vi "DAQ.Get Number of Channels from Channel String.vi"(3 "Channels String":string="PXI1Slot2/ai1:3") -> (1 "# channels":i32)   [LabVIEW 2019, in "Instrument.Lockin.lvlib" / "Instrument.DAQ.lvclass"]
uses:
  Instrument.DAQ.lvclass
panel:
  out "names out":string[](array[string])
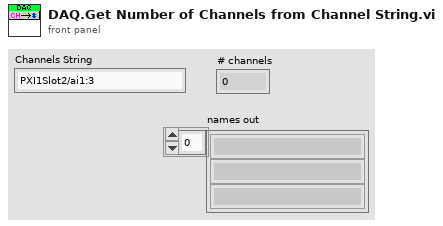
[diagram p1: front panel]
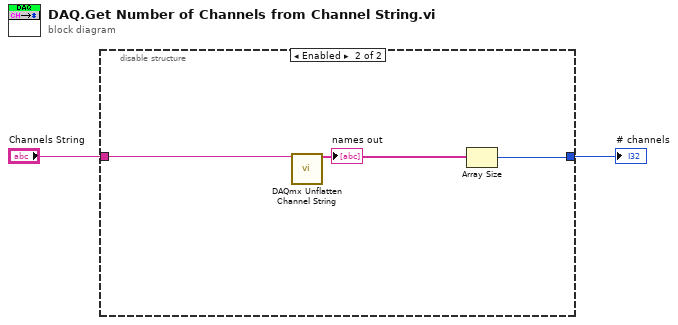
[diagram p0: block diagram]
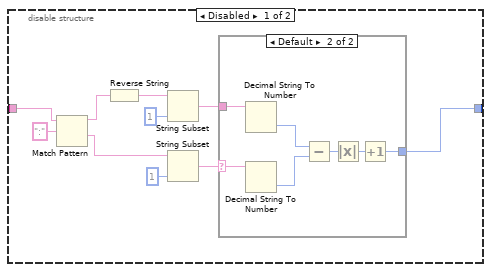
[diagram p2: hidden frame]
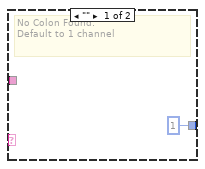
[diagram p3: hidden frame]
diagram:
  n1 = disable-structure shown="Enabled" {
    disable-tunnel: [w5 w21] -> w2
    disable-tunnel: "Channels String" -> [w3 w23]
    frame Disabled {
      n2 = Match Pattern(string=w3, regular expression=":") -> (before substring=w7:string, after substring=w8:string)  [unwired: 1 in, 2 out]
      n3 = Reverse String(1:w7) -> (0:w6:string)
      n4 = String Subset(string=w6, length (rest)=1 ("length (rest)")) -> (substring=w9:string)  [unwired: 1 in]
      n5 = String Subset(string=w8, length (rest)=1 ("length (rest)")) -> (substring=w4:string)  [unwired: 1 in]
      n6 = case shown="Default" w4 {
        selector: w4 -> [_ w17]
        tunnel: w9 -> [_ w20]
        tunnel: [1 w18] -> w5
        frame "" {
          # "No Colon Found:\nDefault to 1 channel"
        }
        frame Default {
          n7 = Decimal String To Number(string=w20) -> (number=w14:i32)  [unwired: 2 in, 1 out]
          n8 = Decimal String To Number(string=w17) -> (number=w15:i32)  [unwired: 2 in, 1 out]
          n9 = Subtract(x=w14, y=w15) -> (x-y=w19:i32)
          n10 = Absolute Value(x=w19) -> (abs(x)=w16:i32)
          n11 = Increment(x=w16) -> (x+1=w18:i32)
        }
      }
    }
    frame Enabled {
      n12 = call <vilib>:"DAQmx Unflatten Channel String.vi"("names in"=w23) -> ("names out"=w22:string[])  [unwired: 13 in, 1 out]
      "names out" <- w22
      n13 = Array Size(array=w22) -> (size(s)=w21:i32)
    }
  }
  "# channels" <- w2
